vi "Get Variable Names.vi"(7 "Target (Process)":T1 items=["Process", "User", "Machine"], 8 "Error In":errorcluster) -> (0 "Error Out":errorcluster, 3 "Names[]":string[](array[string]))   [LabVIEW 2019, in "SLL Environment Variable.lvlib"]
doc: "Get the <B>Names[]</B> of environment variables in the <B>Target</B> environment."
uses:
  SLL Environment Variable.lvlib
  _Typedef/Target Environment Enum.ctl
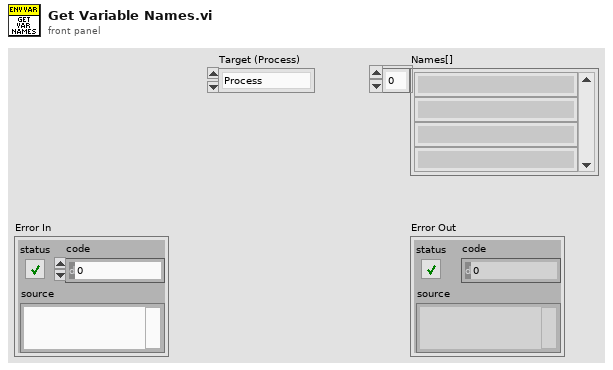
[diagram p1: front panel]
types:
  T1 = typedef "SLL Environment Variable.lvlib/Target Environment Enum.ctl" = i32
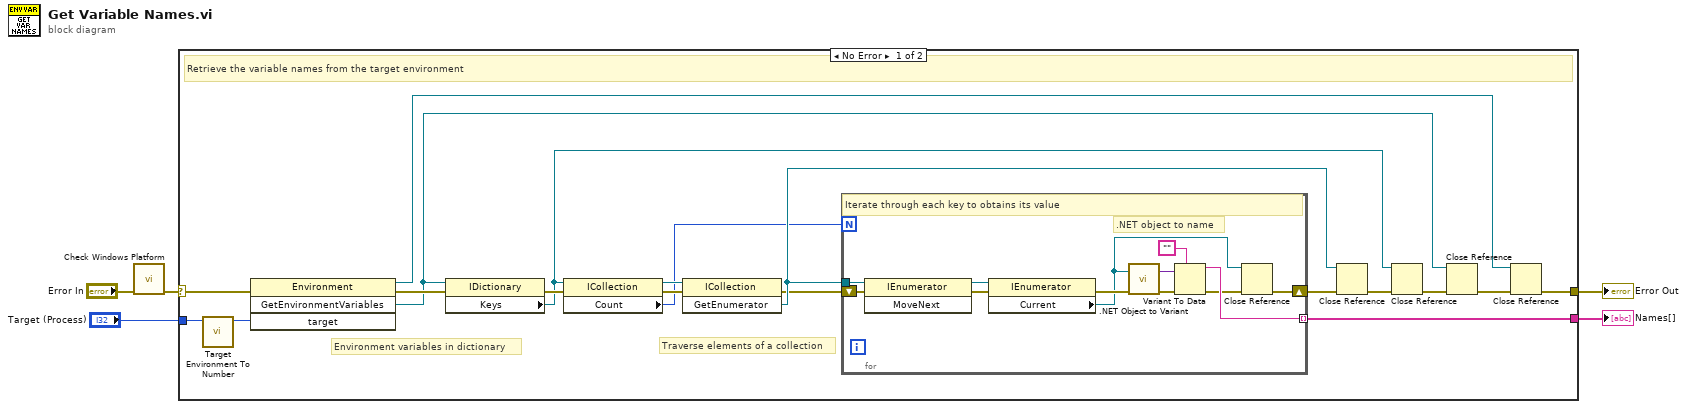
[diagram p0: block diagram]
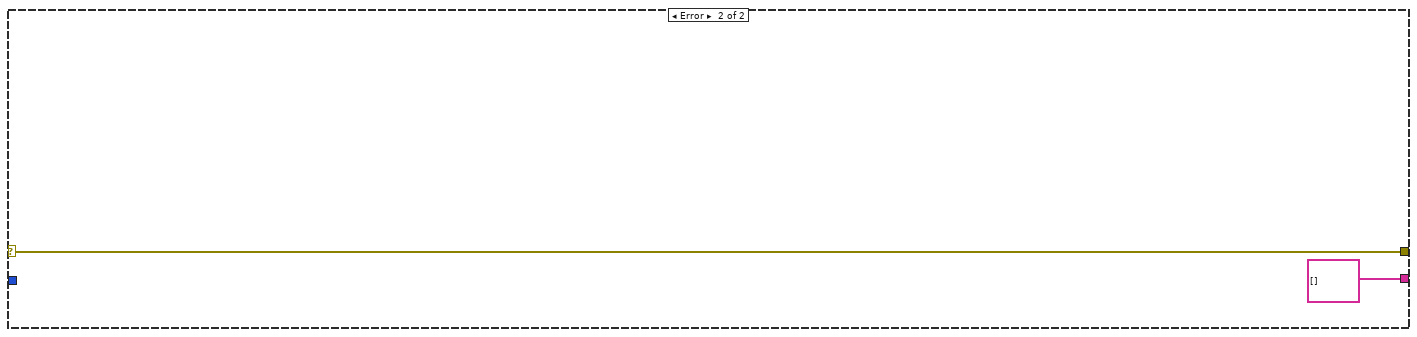
[diagram p2: hidden frame]
diagram:
  n1 = call "Check Windows Platform.vi"("Error In"="Error In") -> ("Error Out"=w2:errorcluster)  [unwired: 10 in]
  n2 = case shown="No Error" w2 {
    selector: w2 -> [w8 w38]
    tunnel: [w13 w38] -> w5
    tunnel: [w9 string[] []] -> w4
    tunnel: "Target (Process)" -> [w7 _]
    frame No Error {
      # "Traverse elements of a collection"
      # "Environment variables in dictionary"
      # "Retrieve the variable names from the target environment"
      n3 = call "Target Environment To Number.vi"("Target (Process)"=w7) -> ("Numeric Value"=w6:i32)  [unwired: 10 in]
      n4 = invoke class="Environment" method="GetEnvironmentVariables"(error in=w8, "target"=w6) -> (reference out=w12:refnum<k24>, error out=w15:errorcluster, "GetEnvironmentVariables"=w14:refnum<k24>)  [unwired: 2 in, 1 out]
      n5 = property class="IDictionary"(reference=w14, error in=w15) -> (error out=w16:errorcluster, "Keys"=w11:refnum<k24>)  [unwired: 1 out]
      n6 = property class="ICollection"(reference=w11, error in=w16) -> (reference out=w18:refnum<k24>, error out=w17:errorcluster, "Count"=w10:i32)
      n7 = invoke class="ICollection" method="GetEnumerator"(reference=w18, error in=w17) -> (error out=w19:errorcluster, "GetEnumerator"=w20:refnum<k24>)  [unwired: 1 in, 1 out]
      n8 = for {
        N: w10 -> [_]
        tunnel: w20 -> [w32]
        tunnel: [w35] -> w9 mode=indexing
        shift-right: [w34] -> w24
        shift-left: w19 -> [w36]
        # ".NET object to name"
        # "Iterate through each key to obtains its value"
        n9 = invoke class="IEnumerator" method="MoveNext"(reference=w32, error in=w36) -> (reference out=w25:refnum<k24>, error out=w33:errorcluster)  [unwired: 1 in, 1 out]
        n10 = property class="IEnumerator"(reference=w25, error in=w33) -> (error out=w31:errorcluster, "Current"=w26:refnum<k24>)  [unwired: 1 out]
        n11 = call <vilib>:".NET Object to Variant.vi"("error in (no error)"=w31, ".NET object"=w26) -> ("error out"=w30:errorcluster, "variant"=w29:variant)
        n12 = Variant To Data(error in=w30, type="", Variant=w29) -> (data=w35:string, error out=w28:errorcluster)
        n13 = Close Reference(reference=w26, error in (no error)=w28) -> (error out=w34:errorcluster)
      }
      n14 = Close Reference(reference=w20, error in (no error)=w24) -> (error out=w21:errorcluster)
      n15 = Close Reference(reference=w11, error in (no error)=w21) -> (error out=w22:errorcluster)
      n16 = Close Reference(reference=w14, error in (no error)=w22) -> (error out=w23:errorcluster)
      n17 = Close Reference(reference=w12, error in (no error)=w23) -> (error out=w13:errorcluster)
    }
    frame Error {
    }
  }
  "Error Out" <- w5
  "Names[]" <- w4
